vi "Main.vi"(11 "Module Admin":refnum<class "Delacor_lib_QMH_Module Admin.lvclass">) -> ()   [LabVIEW 2018, in "DataQuery.lvlib"]
doc: "This template is based off of the Queued Message Handler design pattern and the Queued Message Handler project template that ships with LabVIEW.\n\nThe main difference is that the queue is private to this module and communication between modules is performed via Broadcast and Request events.\n\nRequest events are wrapped in public API methods and are handled in the Event Handling Loop (EHL) of this VI. Any module can register for Broadcast events sent by this module. The EHL generates messages based on user interface actions.\n\nThe Message Handling Loop (MHL) processes messages generated by the EHL, or by other messages. The messages are string values, so new messages can be added easily to the Message Cases case structure in the MHL. Each message cluster can also provide an optional value for Message Data, which is a variant that can be converted to whatever message-specific data is required.\n_____\nBased on DQMH Project Template 6.1.0.94."
uses:
  DataQuery.lvlib
  <vilib>/Delacor/Delacor QMH/Libraries/Module Admin_class/Delacor_lib_QMH_Module Admin.lvclass
  Module Data--cluster.ctl
  <vilib>/Delacor/Delacor QMH/Libraries/Message Queue_class/Delacor_lib_QMH_Message Queue.lvclass/Delacor_lib_QMH_Message Queue.ctl
  Stop Argument--cluster.ctl
  <vilib>/Delacor/Delacor QMH/Libraries/Module Admin_class/Delacor_lib_QMH_Module Admin.lvclass/Delacor_lib_QMH_Module Admin.ctl
  <vilib>/Utility/miscctls.llb/LVPointTypeDef.ctl
  <vilib>/Utility/miscctls.llb/LVMajorAndMinorColorsTypeDef.ctl
  <vilib>/Utility/sysdir.llb/System Directory Type.ctl
  <vilib>/Delacor/Delacor QMH/Libraries/Message Queue_class/Delacor_lib_QMH_Enqueue Message (Single).vi
  <vilib>/Delacor/Delacor QMH/Libraries/Module Admin_class/Delacor_lib_QMH_Get External Launch.vi
  <vilib>/Delacor/Delacor QMH/Libraries/Message Queue_class/Delacor_lib_QMH_Enqueue Message (Array).vi
  <vilib>/Utility/error.llb/Error Cluster From Error Code.vi
  <vilib>/ErrorRing/Error Ring.xnode
  <vilib>/Delacor/Delacor QMH/Libraries/Message Queue_class/Delacor_lib_QMH_Message Queue.lvclass
panel:
  in  "Ring_查询通道":u16(ring) caption="查询通道" items=["ARTM8"]
  in  "Ring_查询日期列表":u16(ring) caption="查询日期文件" items=["20231103-原.tdms", "20231103-温度.tdms", "20231102-温度.tdms"]
  in  "表格/图形":enum32{"table", "graph"}(radio)
  in  "导出曲线":bool
  in  "查询数据":bool
  in  "导出数据":bool
  in  "Ring_查询仪表列表":u16(ring) caption="查询类型" items=["ARTM8"]
  in  "Ring_查询月份列表":u16(ring) caption="查询年月文件夹" items=["负载数据", "2023-11"]
  out "error out":errorcluster
  out "Status":string
  in  "Simulate MHL Error":bool
  in  "Simulate EHL Error":bool
  out "XYGraph":cluster{"时间":dbl[], "数据":dbl[]}(graph) caption="-- 历史曲线"
  in  "Raw data values":i32(listbox) caption="原始数据值"
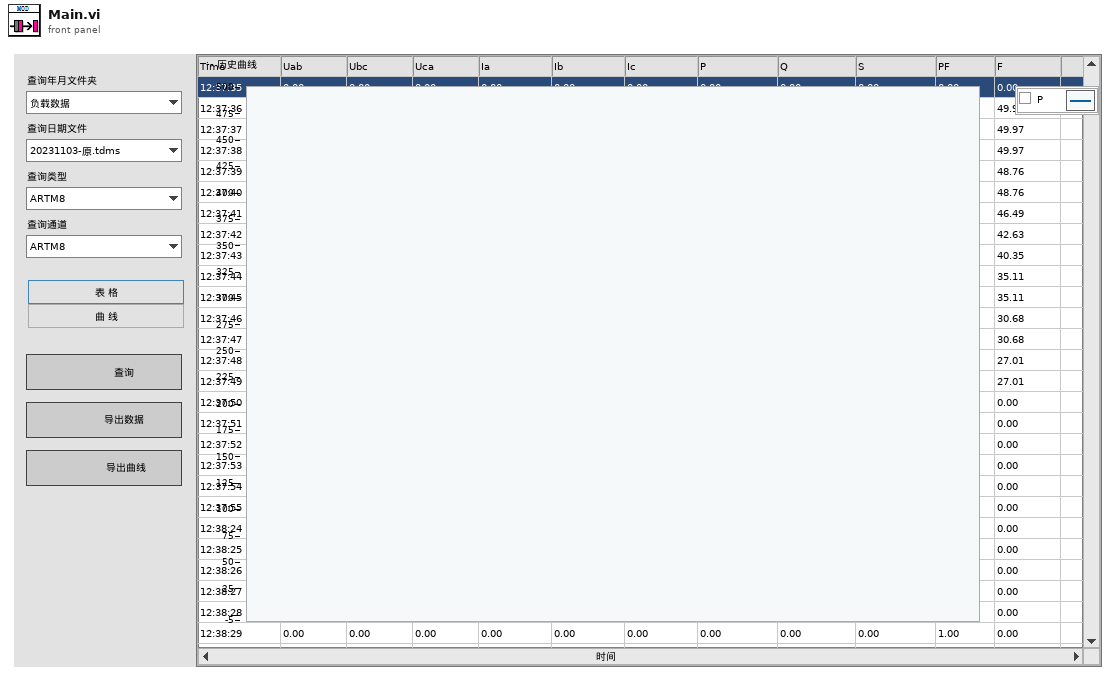
[diagram p1: front panel]
types:
  T1 = typedef "DataQuery.lvlib/Module Data--cluster.ctl" = cluster{"Status":string, "Data Path":path, "Data File":path, "tdms":refnum<k34>}
  T2 = typedef "DataQuery.lvlib/Request Events--cluster.ctl" = cluster{"Stop Module":refnum<user-event>, "Show Panel":refnum<user-event>, "Hide Panel":refnum<user-event>, "Get Module Execution Status":refnum<user-event>, "Show Diagram":refnum<user-event>}
  T3 = enum32{"invalid lock state", "Not Locked", "Locked (No Password)", "Password-protected"}
  T4 = typedef "DataQuery.lvlib/Stop Argument--cluster.ctl" = cluster{"Origin":string, "Exit via Stop Module Req?":bool, "Wait for Module to stop?":bool}
  T5 = enum32{"Invalid", "Standard", "Closed", "Hidden", "Minimized", "Maximized"}
  T6 = enum16{"open", "open or create", "create or replace", "create", "open (read-only)"}
  T7 = typedef "LVPointTypeDef.ctl" = cluster{"Horizontal":i16, "Vertical":i16}
  T8 = typedef "LVMajorAndMinorColorsTypeDef.ctl" = cluster{"Major Color":u32, "Minor Color":u32}
  T9 = typedef "System Directory Type.ctl" = i32
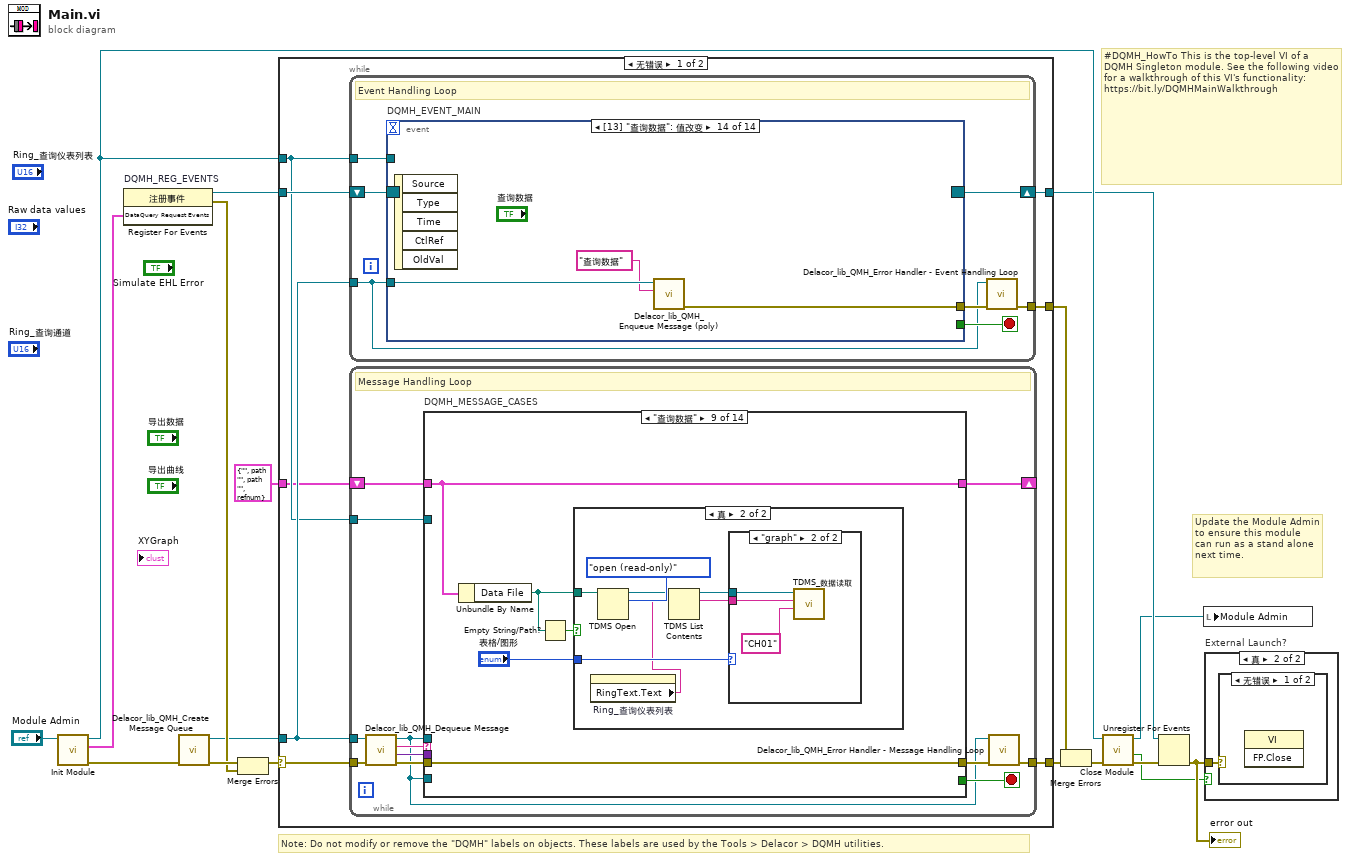
[diagram p0: block diagram]
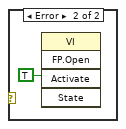
[diagram p3: hidden frame]
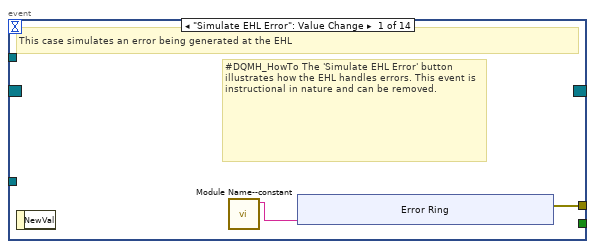
[diagram p4: hidden frame]
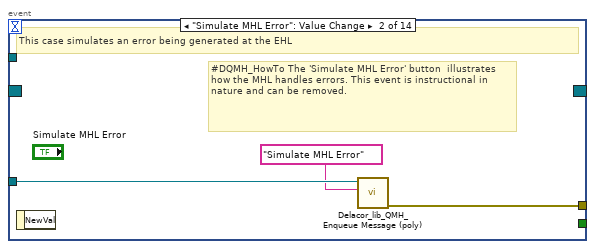
[diagram p5: hidden frame]
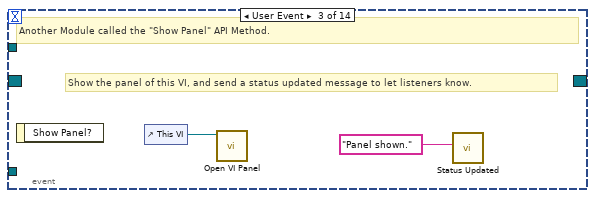
[diagram p6: hidden frame]
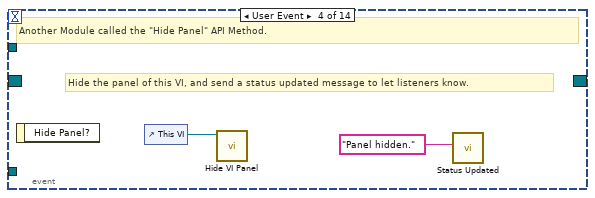
[diagram p7: hidden frame]
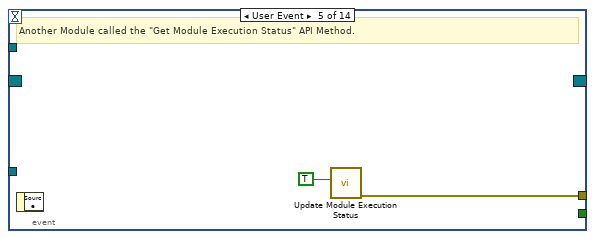
[diagram p8: hidden frame]
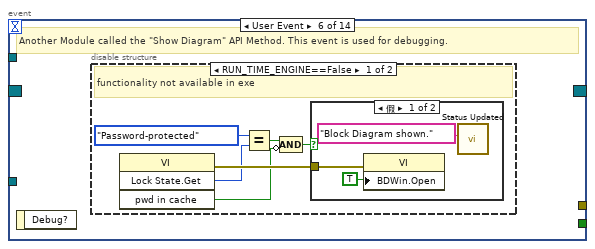
[diagram p9: hidden frame]
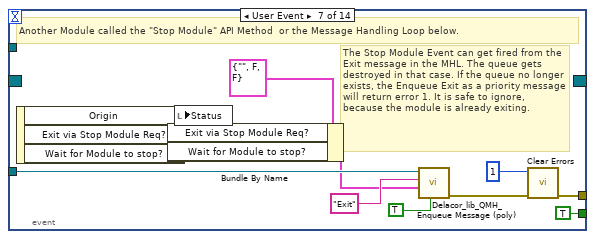
[diagram p12: hidden frame]
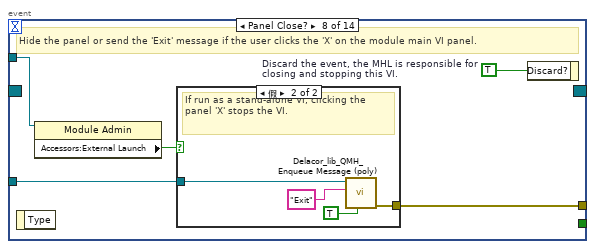
[diagram p13: hidden frame]
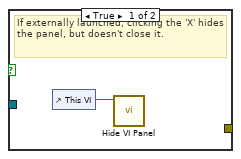
[diagram p14: hidden frame]
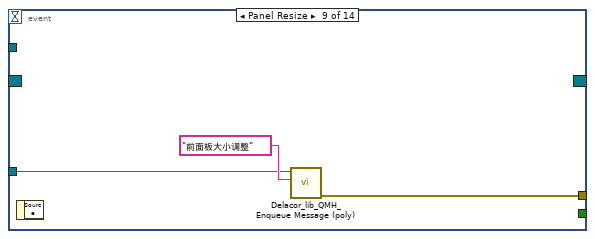
[diagram p15: hidden frame]
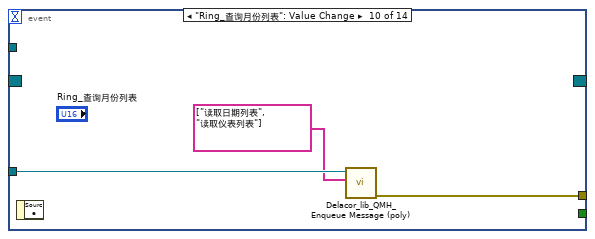
[diagram p16: hidden frame]
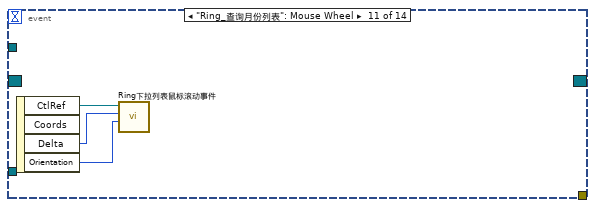
[diagram p17: hidden frame]
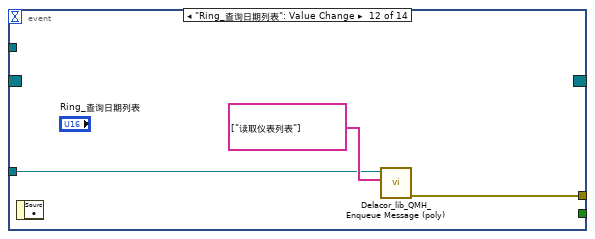
[diagram p18: hidden frame]
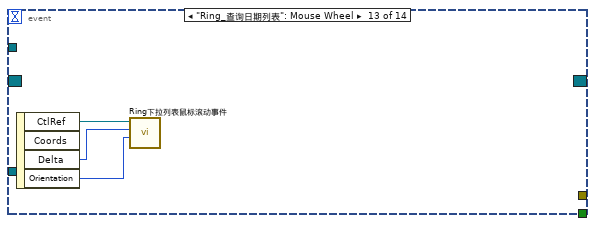
[diagram p19: hidden frame]
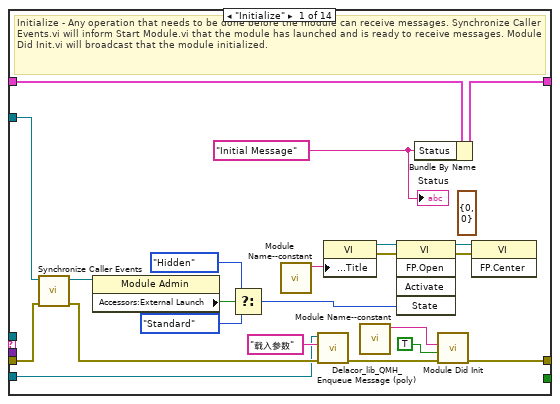
[diagram p20: hidden frame]
diagram:
  # "#DQMH_HowTo This is the top-level VI of a DQMH Singleton module. See the following video for a walkthrough of this VI's functionality: https://bit.ly/DQMHMainWalkthrough"
  # "Note: Do not modify or remove the \"DQMH\" labels on objects. These labels are used by the Tools > Delacor > DQMH utilities."
  # "Update the Module Admin to ensure this module can run as a stand alone next time."
  n1 = call "Init Module.vi"("Singleton Module Admin in"="Module Admin") -> ("error out"=w17:errorcluster, "DataQuery Request Events"=w6:T2, "Singleton Module Admin out"=w9:refnum<class "Delacor_lib_QMH_Module Admin.lvclass">)  [unwired: 8 in]
  n2 = register-events "DQMH_REG_EVENTS"(w6) -> (reference out=w7:refnum<event-registration>, error out=w10:errorcluster)  [unwired: 2 in]
  n3 = call <vilib>:"Delacor_lib_QMH_Create Message Queue.vi"("error in"=w17) -> ("error out"=w12:errorcluster, "Message Queue"=w5:refnum<class "Delacor_lib_QMH_Message Queue.lvclass">)  [unwired: 9 in]
  n4 = Merge Errors(w12, w10) -> (w11:errorcluster)
  n5 = case shown="无错误" w11 {
    selector: w11 -> [w24 w278]
    tunnel: [w26 w277] -> w18
    tunnel: [w23 w283] -> w8
    tunnel: w7 -> [w22 w283]
    tunnel: w5 -> [w21 w276]
    tunnel: [w25 _] -> w15
    tunnel: w9 -> [w20 w279]
    tunnel: T1 {"Status"="", "Data Path"=path "", "Data File"=path "", "tdms"=refnum} ("Data Cluster") -> [w19 _]
    frame No Error {
      n6 = while {
        tunnel: w21 -> [w27]
        shift-right: [w30] -> w23
        shift-left: w22 -> [w31]
        tunnel: [w32] -> w25
        tunnel: w20 -> [w28]
        stop <- w29 stop-if-true
        # "Event Handling Loop"
        n7 = event "DQMH_EVENT_MAIN" shown="[13] \"查询数据\": 值改变" {
          selector: w31 -> [_ _ _ _ _ _ _ _ _ _ _ _ _ _]
          dyn-events: [_ _ _ _ _ _ _ _ _ _ _ _ _ _] -> w30
          timeout: _ -> [_ _ _ _ _ _ _ _ _ _ _ _ _ _]
          tunnel: [_ _ _ _ _ _ TRUE ("Discard?") _ _ _ _ _ _ _] -> w29
          tunnel: w27 -> [_ w44 _ _ _ _ w68 w75 w84 w88 _ w93 _ w100]
          tunnel: [w35 w45 _ _ w51 _ w71 w77 w83 w87 _ w92 _ w99] -> w33
          tunnel: w28 -> [_ _ _ _ _ _ _ w74 _ _ _ _ _ _]
          event "Simulate EHL Error": Value Change {
            # "#DQMH_HowTo The 'Simulate EHL Error' button  illustrates how the EHL handles errors. This event is instructional in nature and can be removed."
            # "This case simulates an error being generated at the EHL"
            n8 = event-data() -> ()  [unwired: 1 in, 1 out]
            n9 = call "Module Name--constant.vi"() -> ("Module Name"=w34:string)  [unwired: 11 in]
            n10 = xnode "Error Ring"("参数 0"=w34) -> ("错误输出"=w35:errorcluster)
          }
          event "Simulate MHL Error": Value Change {
            # "#DQMH_HowTo The 'Simulate MHL Error' button  illustrates how the MHL handles errors. This event is instructional in nature and can be removed."
            # "This case simulates an error being generated at the EHL"
            n11 = event-data() -> ()  [unwired: 1 in, 1 out]
            n12 = call-poly <vilib>:"Delacor_lib_QMH_Enqueue Message (poly).vi"("Message"="Simulate MHL Error", "Message Queue in"=w44) -> ("error out"=w45:errorcluster)  [unwired: 8 in, 1 out]
          }
          event User Event {
            # "Show the panel of this VI, and send a status updated message to let listeners know."
            # "Another Module called the \"Show Panel\" API Method."
            n13 = event-data() -> ()  [unwired: 1 in, 1 out]
            n14 = control-ref of="This VI"() -> (w47:refnum<vi>)
            n15 = call "Open VI Panel.vi"("VI"=w47) -> ()  [unwired: 10 in, 1 out]
            n16 = call "Status Updated.vi"("Status"="Panel shown." ("format string")) -> ()  [unwired: 10 in, 1 out]
          }
          event User Event {
            # "Hide the panel of this VI, and send a status updated message to let listeners know."
            # "Another Module called the \"Hide Panel\" API Method."
            n17 = event-data() -> ()  [unwired: 1 in, 1 out]
            n18 = control-ref of="This VI"() -> (w49:refnum<vi>)
            n19 = call "Hide VI Panel.vi"("VI"=w49) -> ()  [unwired: 10 in, 1 out]
            n20 = call "Status Updated.vi"("Status"="Panel hidden." ("format string")) -> ()  [unwired: 10 in, 1 out]
          }
          event User Event {
            # "Another Module called the \"Get Module Execution Status\" API Method."
            n21 = event-data() -> ()  [unwired: 1 in, 1 out]
            n22 = call "Update Module Execution Status.vi"("Running?"=TRUE) -> ("error out"=w51:errorcluster)  [unwired: 10 in]
          }
          event User Event {
            # "Another Module called the \"Show Diagram\" API Method. This event is used for debugging."
            n23 = event-data() -> ()  [unwired: 1 in, 1 out]
            n24 = disable-structure shown="RUN_TIME_ENGINE==False" {
              frame condition #0 (active) {
                # "functionality not available in exe"
                n25 = invoke class="VI" method="Lock State.Get"() -> (error out=w57:errorcluster, "Get Lock State"=w56:T3, "pwd in cache"=w53:bool)  [unwired: 4 in, 1 out]
                n26 = Equal?(x=T3."Password-protected", y=w56) -> (x = y?=w54:bool)
                n27 = Compound Arithmetic op=AND(w54, invert w53) -> (w52:bool)
                n28 = case "条件结构" shown="假" w52 {
                  tunnel: w57 -> [w60 _]
                  frame False {
                    n29 = property class="VI"(error in=w60, "BDWin.Open"=TRUE ("Block Diagram Window:Open")) -> ()  [unwired: 1 in, 2 out]
                    n30 = call "Status Updated.vi"("Status"="Block Diagram shown." ("format string")) -> ()  [unwired: 10 in, 1 out]
                  }
                  frame True {
                    # "Password-protected VI, and the password is not in the cache. Do not show the diagram."
                  }
                }
              }
              frame condition #1 {
              }
            }
          }
          event User Event {
            # "The Stop Module Event can get fired from the Exit message in the MHL. The queue gets destroyed in that case. If the queue no longer exists, the Enqueue Exit as a priority message will return error 1. It is safe to ignore, because the module is already exiting."
            # "Another Module called the \"Stop Module\" API Method  or the Message Handling Loop below."
            n31 = event-data() -> ("Origin"=w67:string, "Exit via Stop Module Req?"=w63:bool, "Wait for Module to stop?"=w62:bool)  [unwired: 1 in]
            n32 = Bundle By Name(cluster=T4 {"Origin"="", "Exit via Stop Module Req?"=FALSE, "Wait for Module to stop?"=FALSE} ("Stop Argument"), "Exit via Stop Module Req?"=w63, "Wait for Module to stop?"=w62) -> (w61:T4)
            n33 = local write "Status"(w67) -> ()
            n34 = call-poly <vilib>:"Delacor_lib_QMH_Enqueue Message (poly).vi"("Priority Message? (F)"=TRUE, "Message Data"=w61, "Message"="Exit", "Message Queue in"=w68) -> ("error out"=w72:errorcluster)  [unwired: 6 in, 1 out]
            n35 = call <vilib>:"Clear Errors.vi"("error in (no error)"=w72, "specific error code to clear (0: all)"=1) -> ("error out"=w71:errorcluster)  [unwired: 4 in, 1 out]
          }
          event Panel Close? {
            w76 = TRUE  # Discard the event, the MHL is responsible for closing and stopping this VI.
            # "Hide the panel or send the 'Exit' message if the user clicks the 'X' on the module main VI panel."
            n36 = event-data() -> ()  [unwired: 1 in, 1 out]
            n37 = property class="Module Admin"(reference=w74) -> ("Accessors:External Launch"=w73:bool)  [unwired: 1 in, 2 out]
            n38 = case "条件结构" shown="假" w73 {
              tunnel: w75 -> [_ w81]
              tunnel: [_ w82] -> w77
              frame True {
                # "If externally launched, clicking the 'X' hides the panel, but doesn't close it."
                n39 = control-ref of="This VI"() -> (w78:refnum<vi>)
                n40 = call "Hide VI Panel.vi"("VI"=w78) -> ()  [unwired: 10 in, 1 out]
              }
              frame False {
                # "If run as a stand-alone VI, clicking the panel 'X' stops the VI."
                n41 = call-poly <vilib>:"Delacor_lib_QMH_Enqueue Message (poly).vi"("Priority Message? (F)"=TRUE, "Message"="Exit", "Message Queue in"=w81) -> ("error out"=w82:errorcluster)  [unwired: 7 in, 1 out]
              }
            }
            n42 = event-data("Discard?"=w76) -> ()  [unwired: 1 in, 1 out]
          }
          event Panel Resize {
            n43 = event-data() -> ()  [unwired: 1 in, 1 out]
            n44 = call-poly <vilib>:"Delacor_lib_QMH_Enqueue Message (poly).vi"("Message"="前面板大小调整", "Message Queue in"=w84) -> ("error out"=w83:errorcluster)  [unwired: 8 in, 1 out]
          }
          event "Ring_查询月份列表": Value Change {
            n45 = event-data() -> ()  [unwired: 1 in, 1 out]
            n46 = call-poly <vilib>:"Delacor_lib_QMH_Enqueue Message (poly).vi"("Message Array"=string[] ["读取日期列表", "读取仪表列表"] ("Message"), "Message Queue in"=w88) -> ("error out"=w87:errorcluster)  [unwired: 8 in, 1 out]
          }
          event "Ring_查询月份列表": Mouse Wheel {
            n47 = event-data() -> ("CtlRef"=w91:refnum<vi>, "Delta"=w90:i32, "Orientation"=w89:enum16{"Horizontal", "Vertical"})  [unwired: 1 in, 1 out]
            n48 = call "Ring下拉列表鼠标滚动事件.vi"("方向"=w89, "Delta"=w90, "CtlRef"=w91) -> ()  [unwired: 7 in, 2 out]
          }
          event "Ring_查询日期列表": Value Change {
            n49 = event-data() -> ()  [unwired: 1 in, 1 out]
            n50 = call-poly <vilib>:"Delacor_lib_QMH_Enqueue Message (poly).vi"("Message Array"=string[] ["读取仪表列表"] ("Message"), "Message Queue in"=w93) -> ("error out"=w92:errorcluster)  [unwired: 8 in, 1 out]
          }
          event "Ring_查询日期列表": Mouse Wheel {
            n51 = event-data() -> ("CtlRef"=w97:refnum<vi>, "Delta"=w96:i32, "Orientation"=w95:enum16{"Horizontal", "Vertical"})  [unwired: 1 in, 1 out]
            n52 = call "Ring下拉列表鼠标滚动事件.vi"("方向"=w95, "Delta"=w96, "CtlRef"=w97) -> ()  [unwired: 7 in, 2 out]
          }
          event "查询数据": Value Change {
            n53 = event-data() -> ()  [unwired: 1 in, 5 out]
            n54 = call-poly <vilib>:"Delacor_lib_QMH_Enqueue Message (poly).vi"("Message"="查询数据", "Message Queue in"=w100) -> ("error out"=w99:errorcluster)  [unwired: 8 in, 1 out]
          }
        }
        n55 = call-dynamic "Delacor_lib_QMH_Error Handler - Event Handling Loop.vi"("error in"=w33, "Message Queue in"=w27) -> ("dup error in"=w32:errorcluster)  [unwired: 8 in, 1 out]
      }
      n56 = while {
        tunnel: w21 -> [w103]
        shift-right: [w107] -> _
        shift-left: w19 -> [w108]
        tunnel: w24 -> [w111]
        tunnel: [w109] -> w26
        tunnel: w20 -> [w102]
        stop <- w106 stop-if-true
        # "Message Handling Loop"
        n57 = call-dynamic "Delacor_lib_QMH_Dequeue Message.vi"("error in"=w111, "Message Queue in"=w103) -> ("error out"=w110:errorcluster, "Message Data"=w104:variant, "Message"=w105:string, "Message Queue out"=w101:refnum<class "Delacor_lib_QMH_Message Queue.lvclass">)  [unwired: 6 in]
        n58 = case "DQMH_MESSAGE_CASES" shown="\"查询数据\"" w105 {
          selector: w105 -> [_ _ _ _ _ _ _ _ _ _ _ _ _ w263]
          tunnel: w101 -> [_ w138 _ _ _ _ _ _ _ _ _ w233 w255 _]
          tunnel: w110 -> [w132 w137 w150 w153 w155 w169 w180 w195 w206 w218 w223 w240 w261 w265]
          tunnel: [w131 w136 w150 w152 w155 w169 w180 w195 w206 w218 w222 w236 w258 w266] -> w112
          tunnel: w108 -> [w122 w148 w149 w151 w154 w168 w179 w191 w205 w217 w220 w235 w254 w264]
          tunnel: [w121 w148 w149 w151 w154 w157 w179 w185 w205 w217 w220 w235 w254 w264] -> w107
          tunnel: [_ _ _ _ _ _ _ _ _ _ _ _ w253 _] -> w106
          tunnel: w104 -> [_ _ _ _ _ _ _ _ _ _ _ w234 w252 _]
          tunnel: w102 -> [w123 _ _ _ _ _ _ _ _ _ _ w232 w247 _]
          tunnel: w101 -> [w113 _ _ _ _ _ _ _ _ _ _ _ _ _]
          frame "Initialize" {
            (unwired) T7 {"Horizontal"=0, "Vertical"=0} ("Origin")
            w117 = "Initial Message" ("Initial Message")
            # "Initialize - Any operation that needs to be done before the module can receive messages. Synchronize Caller Events.vi will inform Start Module.vi that the module has launched and is ready to receive messages. Module Did Init.vi will broadcast that the module initialized."
            n59 = call "Synchronize Caller Events.vi"("error in (no error)"=w132, "Singleton Module Admin in"=w123) -> ("error out"=w116:errorcluster, "Singleton Module Admin out"=w118:refnum<class "Delacor_lib_QMH_Module Admin.lvclass">)  [unwired: 8 in]
            n60 = property class="Module Admin"(reference=w118) -> ("Accessors:External Launch"=w127:bool)  [unwired: 1 in, 2 out]
            n61 = Select(t=T5."Hidden" ("State"), s=w127, f=T5."Standard" ("State")) -> (s? t:f=w124:T5)
            n62 = call "Module Name--constant.vi"() -> ("Module Name"=w130:string)  [unwired: 11 in]
            n63 = call-poly <vilib>:"Delacor_lib_QMH_Enqueue Message (poly).vi"("error in"=w116, "Message"="载入参数", "Message Queue in"=w113) -> ("error out"=w115:errorcluster)  [unwired: 7 in, 1 out]
            n64 = property class="VI"("Front Panel.Title"=w130) -> (reference out=w129:refnum<vi>, error out=w134:errorcluster)  [unwired: 2 in]
            n65 = call "Module Name--constant.vi"() -> ("Module Name"=w119:string)  [unwired: 11 in]
            n66 = invoke class="VI" method="FP.Open"(reference=w129, error in=w134, "State"=w124) -> (reference out=w128:refnum<vi>, error out=w133:errorcluster)  [unwired: 2 in, 3 out]
            n67 = Bundle By Name(cluster=w122, "Status"=w117) -> (w121:T1)
            n68 = call "Module Did Init.vi"("error in (no error)"=w115, "Initialized?"=TRUE, "Origin"=w119) -> ("error out"=w131:errorcluster)  [unwired: 8 in]
            n69 = invoke class="VI" method="FP.Center"(reference=w128, error in=w133) -> ()  [unwired: 1 in, 3 out]
            "Status" <- w117
          }
          frame "载入参数" {
            w145 = T8 {"Major Color"=16777216, "Minor Color"=16777216}  # 无网格
            n70 = control-ref of="XYGraph"() -> (w139:refnum<vi>)
            n71 = call <vilib>:"Application Directory.vi"() -> ("Application Directory"=w147:path)
            n72 = Build Path(base path=w147, name or relative path=".\\data\\Config.ini" ("名称或相对路径")) -> ()  [unwired: 1 out]
            n73 = call-poly <vilib>:"Delacor_lib_QMH_Enqueue Message (poly).vi"("error in"=w137, "Message Array"=string[] ["读取年月列表", "读取日期列表", "读取仪表列表"] ("Message"), "Message Queue in"=w138) -> ("error out"=w136:errorcluster)  [unwired: 7 in, 1 out]
            n74 = property on="属性节点" class="XYGraph (严格)"(reference=w139, "XScale.GridColors"=w145, "YScale.GridColors"=w145, "YScale.Maximum"=500.0 ("Y标尺.范围:最大值"), "YScale.Minimum"=-5.0 ("Y标尺.范围:最小值"), "XScale.NameLbl.Text"="时间" ("X标尺.名称标签.文本"), "YScale.NameLbl.Text"="幅值" ("Y标尺.名称标签.文本"), "Caption.Text"="   -- 历史曲线" ("标题.文本")) -> ()  [unwired: 1 in, 2 out]
            n75 = call "窗格_所有窗格居中显示.vi"() -> ()  [unwired: 11 in, 1 out]
          }
          frame "---Module Specific---" {
            # "Separator -- The following cases handle messages specific to this Module."
          }
          frame "---Copy This Frame---" {
            # "Duplicate this frame when creating new messages.  Change this comment in the duplicated frame to describe this message."
            n76 = Merge Errors(w153) -> (w152:errorcluster)
          }
          frame "前面板大小调整" {
            n77 = call "Table_根据窗格自动缩放.vi"() -> ()  [unwired: 11 in, 1 out]
          }
          frame "读取年月列表" {
            w167 = T9 1 items=["用户目录"=0, "用户桌面"=1, "用户文档"=2, "用户应用程序数据"=3, "用户设置"=4, "用户临时目录"=5, "公共文档"=6, "公共应用程序数据"=7, "公共设置"=8, "公共缓存"=13, "系统核心库"=9, "系统安装库"=10, "应用程序文件"=11, "启动盘根目录"=12] ("system directory type")
            n78 = call <vilib>:"Get System Directory.vi"("system directory type"=w167) -> ("system directory"=w166:path)  [unwired: 10 in]
            n79 = Build Path(base path=w166, name or relative path="LB Data" ("名称或相对路径")) -> (appended path=w156:path)
            n80 = List Folder(path=w156) -> (folder names=w159:string[])  [unwired: 3 in, 3 out]
            n81 = control-ref of="Ring_查询月份列表"() -> (w164:refnum<vi>)
            n82 = Search 1D Array(1D array=w159, element="DataBase" ("元素")) -> (index of element=w160:i32)  [unwired: 1 in]
            n83 = Delete From Array(array=w159, index=w160) -> (array with subset deleted=w158:string[])  [unwired: 1 in, 1 out]
            n84 = Reverse 1D Array(array=w158) -> (reversed array=w163:string[])
            n85 = Bundle By Name(cluster=w168, "Data Path"=w156) -> (w157:T1)
            n86 = property class="Ring (严格)"(reference=w164, "Strings []"=w163, "Value"=u16 0 ("值")) -> ()  [unwired: 1 in, 2 out]
          }
          frame "读取日期列表" {
            n87 = control-ref of="Ring_查询月份列表"() -> (w177:refnum<vi>)
            n88 = Unbundle By Name(w179) -> ("Data Path"=w178:path)
            n89 = property class="Ring (严格)"(reference=w177) -> ("RingText.Text"=w176:string)  [unwired: 1 in, 2 out]
            n90 = control-ref of="Ring_查询日期列表"() -> (w173:refnum<vi>)
            n91 = Build Path(base path=w178, name or relative path=w176) -> (appended path=w172:path)
            n92 = List Folder(path=w172, pattern="*.tdms" ("类型")) -> (filenames=w170:string[])  [unwired: 2 in, 3 out]
            n93 = Reverse 1D Array(array=w170) -> (reversed array=w175:string[])
            n94 = property class="Ring (严格)"(reference=w173, "Strings []"=w175, "Value"=u16 0 ("值")) -> ()  [unwired: 1 in, 2 out]
          }
          frame "读取仪表列表" {
            n95 = control-ref of="Ring_查询日期列表"() -> (w190:refnum<vi>)
            n96 = control-ref of="Ring_查询月份列表"() -> (w193:refnum<vi>)
            n97 = Unbundle By Name(w191) -> ("Data Path"=w194:path)
            n98 = property class="Ring (严格)"(reference=w190) -> ("RingText.Text"=w188:string)  [unwired: 1 in, 2 out]
            n99 = property class="Ring (严格)"(reference=w193) -> ("RingText.Text"=w192:string)  [unwired: 1 in, 2 out]
            n100 = Build Path(base path=w194, name or relative path=w192) -> (appended path=w189:path)
            n101 = Build Path(base path=w189, name or relative path=w188) -> (appended path=w184:path)
            n102 = call <vilib>:"Check if File or Folder Exists.vi"("path"=w184) -> ("file or folder exists?"=w187:bool, "dup path"=w186:path)  [unwired: 8 in, 1 out]
            n103 = case shown="真" w187 {
              tunnel: w186 -> [_ w197]
              tunnel: [_ w198] -> w183
              tunnel: [path "" w197] -> w181
              frame False {
              }
              frame True {
                n104 = TDMS Open(10:T6."open (read-only)" ("操作(0:open)"), 11:w197) -> (3:w200:refnum<k34>)  [unwired: 5 in, 1 out]
                n105 = TDMS List Contents(7:w200) -> (2:w198:string[], 3:w199:refnum<k34>)  [unwired: 2 in, 2 out]
                n106 = TDMS Close(11:w199) -> ()  [unwired: 1 in, 2 out]
              }
            }
            n107 = property on="Ring_查询仪表列表" class="Ring (严格)"("Strings []"=w183, "Value"=0) -> ()  [unwired: 2 in, 2 out]
            n108 = Bundle By Name(cluster=w191, "Data File"=w181) -> (w185:T1)
          }
          frame "查询数据" {
            n109 = Unbundle By Name(w205) -> ("Data File"=w203:path)
            n110 = Empty String/Path?(string/path=w203) -> (empty?=w204:bool)
            n111 = case shown="真" w204 {
              tunnel: w203 -> [_ w213]
              tunnel: "表格/图形" -> [_ w211]
              frame False {
              }
              frame True {
                n112 = property on="Ring_查询仪表列表" class="Ring (严格)"() -> ("RingText.Text"=w208:string)  [unwired: 2 in, 2 out]
                n113 = TDMS Open(10:T6."open (read-only)" ("操作(0:open)"), 11:w213) -> (3:w210:refnum<k34>)  [unwired: 5 in, 1 out]
                n114 = TDMS List Contents(6:w208, 7:w210) -> (2:w207:string, 3:w209:refnum<k34>)  [unwired: 1 in, 2 out]
                n115 = case shown="\"graph\"" w211 {
                  tunnel: w209 -> [_ w216]
                  tunnel: w207 -> [_ w214]
                  frame "table", Default {
                  }
                  frame "graph" {
                    n116 = call "TDMS_数据读取.vi"("CH Name[]"="CH01", "组名称"=w214, "tdms文件"=w216) -> ()  [unwired: 4 in, 5 out]
                  }
                }
              }
            }
          }
          frame "---Exit and Error Handling---" {
            # "Separator - The following cases handle errors and exit messages."
          }
          frame "Simulate MHL Error" {
            # "#DQMH_HowTo The 'Simulate MHL Error' button  illustrates how the MHL handles errors. This event is instructional in nature and can be removed."
            # "Simulate an error occurring at the MHL"
            n117 = call "Module Name--constant.vi"() -> ("Module Name"=w219:string)  [unwired: 11 in]
            n118 = xnode "Error Ring"("参数 0"=w219) -> ("错误输出"=w221:errorcluster)
            n119 = Merge Errors(w223, w221) -> (w222:errorcluster)
          }
          frame "Error" {
            # "#CodeRecommended - If you ever change the name of this \"Error\" message, you'll need to update the name in the Check Loop Error.vi as well."
            # "#CodeRecommended - If the module is running in standalone mode (External Launch = FALSE), this code will pop up an error dialog and call the 'Exit' message if an error occurs. Add more fine-grained error handling here."
            # "Error - Check the error message data and respond accordingly. This message is sent by the \"Error Handler\" VIs at the end of each loop in this application."
            n120 = property class="Module Admin"(reference=w232) -> ("Accessors:External Launch"=w231:bool)  [unwired: 1 in, 2 out]
            n121 = Variant To Data(error in=w240, type=errorcluster {"status"=FALSE, "code"=0, "source"=""} ("error constant"), Variant=w234) -> (data=w241:errorcluster, error out=w238:errorcluster)
            n122 = call "Error Reported.vi"("Error"=w241) -> ()  [unwired: 10 in, 1 out]
            n123 = case shown="假" w231 {
              tunnel: [w246 _] -> w237
              tunnel: w233 -> [w244 _]
              tunnel: w241 -> [w245 _]
              frame False {
                # "If the module is running standalone, then pop up an error dialog and call the \"Exit\" message."
                n124 = call <vilib>:"Simple Error Handler.vi"("error in (no error)"=w245) -> ()  [unwired: 4 in, 5 out]
                n125 = call-poly <vilib>:"Delacor_lib_QMH_Enqueue Message (poly).vi"("Priority Message? (F)"=TRUE, "Message"="Exit", "Message Queue in"=w244) -> ("error out"=w246:errorcluster)  [unwired: 7 in, 1 out]
              }
              frame True {
                # "If the module was launched externally, calling the Error Reported broadcast VI is the only action performed by the \"Error\" message. The module's caller can then process the error appropriately."
              }
            }
            n126 = Merge Errors(w238, w237) -> (w236:errorcluster)
            n127 = local write "error out"(w236) -> ()
          }
          frame "Exit" {
            w251 = 91  # 91: not all Exit messages will have an argument
            w253 = TRUE  # Stop the VI
            # "Release the message queue reference"
            # "#CodeNeeded - Add any required cleanup code here"
            # "Exit - Exit the application."
            n128 = Variant To Data(error in=w261, type=T4 {"Origin"="", "Exit via Stop Module Req?"=FALSE, "Wait for Module to stop?"=FALSE} ("Stop Argument"), Variant=w252) -> (data=w249:T4, error out=w257:errorcluster)
            n129 = call <vilib>:"Clear Errors.vi"("error in (no error)"=w257, "specific error code to clear (0: all)"=w251) -> ("error out"=w260:errorcluster)  [unwired: 4 in, 1 out]
            n130 = control-ref of="This VI"() -> (w248:refnum<vi>)
            n131 = call-dynamic "Delacor_lib_QMH_Release Message Queue.vi"("error in"=w260, "Message Queue"=w255) -> ("error out"=w259:errorcluster)  [unwired: 9 in]
            n132 = call "Handle Exit.vi"("Stop Argument"=w249, "Admin in"=w247, "VI reference"=w248) -> ("error out"=w256:errorcluster)  [unwired: 7 in, 1 out]
            n133 = Merge Errors(w259, w256) -> (w258:errorcluster)
          }
          frame Default {
            # "'Default' case only runs if there is a message that isn't defined in any of the other cases.  Output a programming error."
            n134 = call "Module Name--constant.vi"() -> ("Module Name"=w262:string)  [unwired: 11 in]
            n135 = xnode "Error Ring"("参数 0"=w263, "参数 1"=w262) -> ("错误输出"=w267:errorcluster)
            n136 = Merge Errors(w265, w267) -> (w266:errorcluster)
          }
        }
        n137 = call-dynamic "Delacor_lib_QMH_Error Handler - Message Handling Loop.vi"("error in"=w112, "Message Queue in"=w101) -> ("dup error in"=w109:errorcluster)  [unwired: 8 in, 1 out]
      }
    }
    frame Error {
      # "Synchronize Caller Events.vi will inform Start Module.vi that the module has launched and will let the code calling Start Module.vi register for broadcasts and would permit the caller receive the broadcast that an error occurred at launch time."
      n138 = call-dynamic "Delacor_lib_QMH_Release Message Queue.vi"("error in"=w278, "Message Queue"=w276) -> ("error out"=w277:errorcluster)  [unwired: 9 in]
      n139 = call "Synchronize Caller Events.vi"("Singleton Module Admin in"=w279) -> ("error out"=w284:errorcluster)  [unwired: 9 in, 1 out]
      n140 = call "Module Name--constant.vi"() -> ("Module Name"=w282:string)  [unwired: 11 in]
      n141 = Format Into String(format string="An error occurred during initialization. %s is no longer running.", w282) -> (resulting string=w280:string)  [unwired: 2 in, 1 out]
      n142 = Merge Errors(w277, w284) -> (w285:errorcluster)
      n143 = call "Error Reported.vi"("Additional Information"=w280, "Error"=w285) -> ()  [unwired: 9 in, 1 out]
    }
  }
  n144 = Merge Errors(w15, w18) -> (w14:errorcluster)
  n145 = call "Close Module.vi"("error in (no error)"=w14, "Module Admin in"=w9) -> ("error out"=w16:errorcluster, "External Launch"=w2:bool, "Module Admin out"=w3:refnum<class "Delacor_lib_QMH_Module Admin.lvclass">)  [unwired: 7 in]
  n146 = Unregister For Events(event registration refnum=w8, error in=w16) -> (error out=w13:errorcluster)
  "error out" <- w13
  n147 = local write "Module Admin"(w3) -> ()
  n148 = case "External Launch?" shown="真" w2 {
    tunnel: w13 -> [_ w286]
    frame False {
    }
    frame True {
      n149 = case "条件结构" shown="无错误" w286 {
        frame No Error {
          n150 = invoke class="VI" method="FP.Close"() -> ()  [unwired: 3 in, 3 out]
        }
        frame Error {
          n151 = invoke class="VI" method="FP.Open"("Activate"=TRUE ("Activate?")) -> ()  [unwired: 4 in, 5 out]
        }
      }
    }
  }
